vi "Send UI Msg.vi"(8 "error in (no error)":errorcluster, 9 "Data":variant, 10 "Msg":T1, 11 "Editor.lvclass in":refnum<data-value>) -> (0 "error out":errorcluster, 3 "Editor.lvclass out":refnum<data-value>)   [LabVIEW 2015, in "Editor.lvclass"]
uses:
  Editor.lvclass
  UI_MSG.ctl
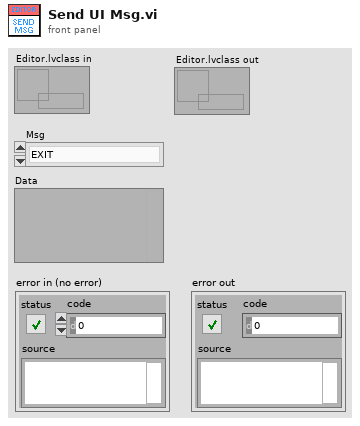
[diagram p1: front panel]
types:
  T1 = typedef "Editor.lvclass/UI_MSG.ctl" = enum16{"EXIT", "INIT_UI", "NEW_PROJECT", "OPEN_PROJECT", "STEP_DISPLAY_UPDATE", "STEP_OPERATION", "UPDATE_UI", "ACTIVE_OBJECT", "DEACTIVE_OBJECT", "SAVE_PROJECT"}
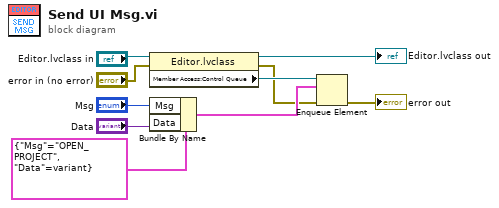
[diagram p0: block diagram]
diagram:
  n1 = property class="Editor.lvclass"(reference="Editor.lvclass in", error in="error in (no error)") -> (reference out=→"Editor.lvclass out":refnum<data-value>, error out=w3:errorcluster, "Member Access:Control Queue"=w4:refnum<queue>)
  n2 = Bundle By Name(cluster=cluster{"Msg":T1, "Data":variant} {"Msg"=enum."OPEN_PROJECT", "Data"=variant}, "Msg"="Msg", "Data"="Data") -> (w8:cluster{"Msg":T1, "Data":variant})
  n3 = Enqueue Element(queue=w4, element=w8, error in (no error)=w3) -> (error out=→"error out":errorcluster)  [unwired: 1 in, 2 out]
